vi "Alphabetize Cluster Elements.vi"(6 "Mouse Position":T1, 7 "User VI Ref":refnum<vi>, 8 "Is Multi-select?":bool, 9 "Remaining Items":refnum<vi>[](array[refnum]), 10 "Affected Items":T8, 11 "Menu Refnum":refnum<k9>) -> (3 "Menu Items To Add":T2[](array[typedef]))   [LabVIEW 2017, in "Shortcut Menu.lvlib"]
doc: "This VI is part of a plug-in for modifying the LabVIEW shortcut menus. This is the builder VI which is called when the shortcut menu is built. It tells LabVIEW which shortcut menu items to add to the menu."
uses:
  Shortcut Menu.lvlib
  <resource>/plugins/PopupMenus/support/Shortcut Menu Item Definition.ctl
  <resource>/plugins/PopupMenus/support/Transaction Control.ctl
  <resource>/plugins/PopupMenus/support/Position In Menu.ctl
  <resource>/plugins/PopupMenus/support/Relative Position.ctl
  <resource>/plugins/PopupMenus/support/Checkmark Status.ctl
  <resource>/plugins/PopupMenus/support/Enabled Menu Item Status.ctl
  Alphabetize Cluster Elements.ctl
  <vilib>/Utility/miscctls.llb/LVPositionTypeDef.ctl
  Toolkit/Toolkit.lvlib
panel:
  # "Rules a popup plug-in must follow:\n* This VI's file name must match the file name of the LLB -- only the file extensions should be different.\n* This VI must have debugging disabled or it will be ignored as a plug-in.\n* For all menu items, \"tag suffix + file name of this VI\" must be less than 240 characters.\n* You can disconnect the \"Affected Items\" from the typedef to make the plug-in load faster. The typedef is only there to assist you in keeping this VI and the execution VI using to the same type.\n* All controls on this panel except \"Affected Items\" are locked to prevent accidental edits. Do not change the types or the names of controls other than the elements inside the \"Affected Items\" cluster.\n* See Context Help for more information on the individual controls."
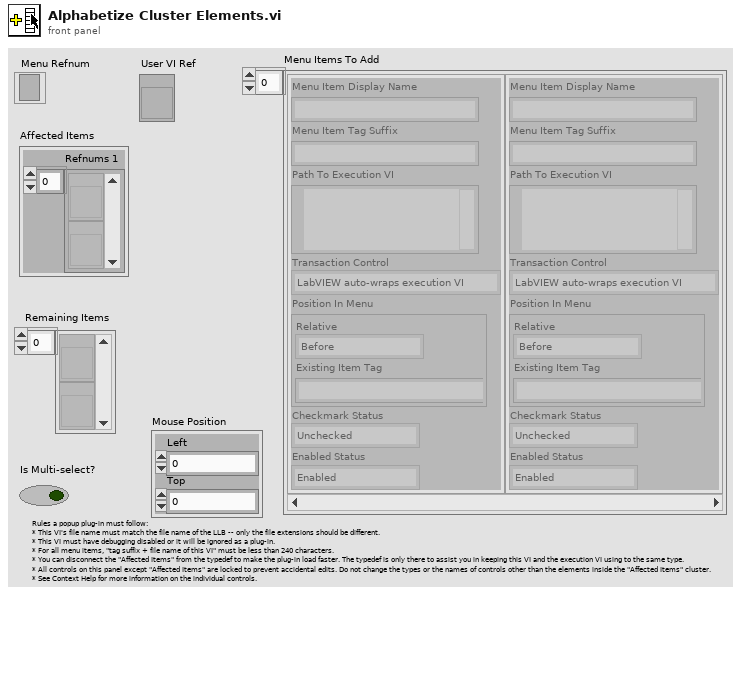
[diagram p1: front panel]
types:
  T1 = typedef "LVPositionTypeDef.ctl" = cluster{"Left":i32, "Top":i32}
  T2 = typedef "Shortcut Menu Item Definition.ctl" = cluster{"Menu Item Display Name":string, "Menu Item Tag Suffix":string, "Path To Execution VI":path, "Transaction Control":T3, "Position In Menu":T4, "Checkmark Status":T6, "Enabled Status":T7}
  T3 = typedef "Transaction Control.ctl" = enum8{"LabVIEW auto-wraps execution VI", "Execution VI will define if needed"}
  T4 = typedef "Position In Menu.ctl" = cluster{"Relative":T5, "Existing Item Tag":string}
  T5 = typedef "Relative Position.ctl" = enum8{"Before", "Instead of", "After", "Into Submenu"}
  T6 = typedef "Checkmark Status.ctl" = enum8{"Unchecked", "Checked"}
  T7 = typedef "Enabled Menu Item Status.ctl" = enum8{"Enabled", "Disabled"}
  T8 = typedef "Alphabetize Cluster Elements.ctl" = cluster{"Refnums 1":refnum<vi>[]}
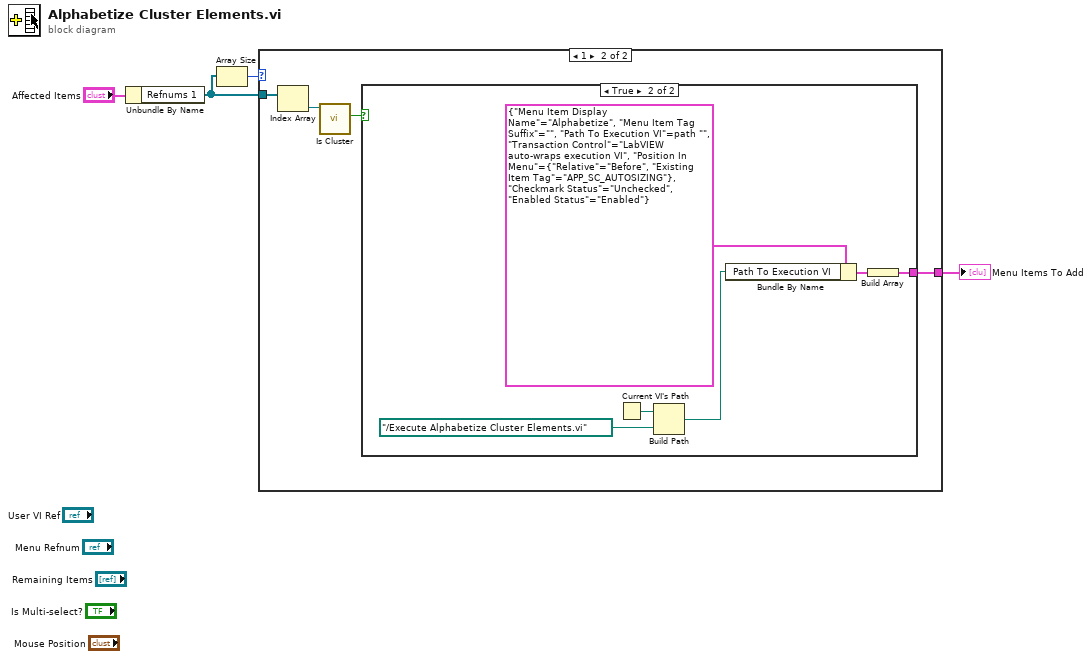
[diagram p0: block diagram]
diagram:
  n1 = Unbundle By Name("Affected Items") -> ("Refnums 1"=w1:refnum<vi>[])
  n2 = Array Size(array=w1) -> (size(s)=w2:i32)
  n3 = case shown="1" w2 {
    tunnel: [_ w8] -> w4
    tunnel: w1 -> [_ w7]
    frame Default {
    }
    frame 1 {
      n4 = Index Array(array=w7) -> (element=w6:refnum<vi>)  [unwired: 1 in]
      n5 = call "Is Cluster.vi"("GObject In"=w6) -> ("Cluster?"=w5:bool)  [unwired: 8 in, 2 out]
      n6 = case shown="True" w5 {
        tunnel: [_ w10] -> w8
        frame False {
        }
        frame True {
          n7 = Current VI's Path() -> (path=w9:path)
          n8 = Build Path(base path=w9, name or relative path=path "../Execute Alphabetize Cluster Elements.vi" ("execute path")) -> (appended path=w13:path)
          n9 = Bundle By Name(cluster=T2 {"Menu Item Display Name"="Alphabetize", "Menu Item Tag Suffix"="", "Path To Execution VI"=path "", "Transaction Control"=enum."LabVIEW auto-wraps execution VI", "Position In Menu"={"Relative"=enum."Before", "Existing Item Tag"="APP_SC_AUTOSIZING"}, "Checkmark Status"=enum."Unchecked", "Enabled Status"=enum."Enabled"} ("Cluster"), "Path To Execution VI"=w13) -> (w11:T2)
          n10 = Build Array(w11) -> (w10:T2[])
        }
      }
    }
  }
  "Menu Items To Add" <- w4
